vi "Set Config (Element).vi"(8 "error in (no error)":errorcluster, 10 "Config Element":refnum<class "Config Element.lvclass">, 11 "Task in":refnum<class "Task.lvclass">) -> (0 "error out":errorcluster, 3 "Task out":refnum<class "Task.lvclass">)   [LabVIEW 2020, in "Volatus.lvlib" / "Task.lvclass"]
uses:
  Task.lvclass
  lv-cdm/CDM-Config/Config Element/Config Element.lvclass
  Task.lvclass/Task.ctl
  VolatusConfig/Task/Task.lvclass
  VolatusConfig/VolatusConfigElement/VolatusConfigElement.lvclass
  C:/dev/lv20CE/relink/lv-volatus/VolatusConfig/VolatusConfigElement/VolatusConfigElement.lvclass
  C:/dev/lv20CE/relink/lv-volatus/VolatusConfig/Task/Task.lvclass
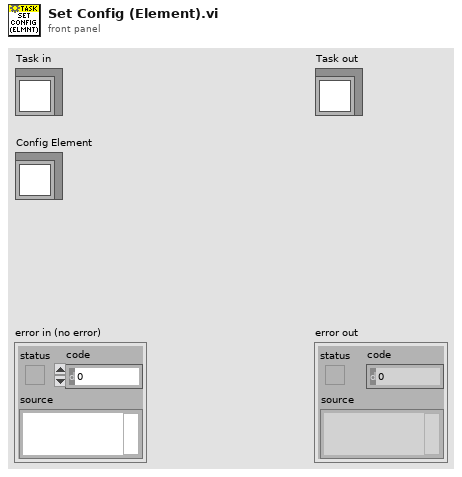
[diagram p1: front panel]
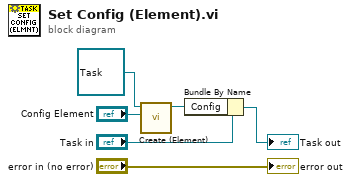
[diagram p0: block diagram]
diagram:
  n1 = call "Create (Element).vi"("Element"="Config Element", "VolatusConfigElement in"=refnum<class "Task.lvclass"> refnum ("VolatusConfig.lvlib:Task.lvclass")) -> ("VolatusConfigElement out"=w2:refnum<class "Task.lvclass">)  [unwired: 8 in, 1 out]
  n2 = Bundle By Name(cluster="Task in", "Config"=w2) -> (→"Task out":refnum<class "Task.lvclass">)
  "error out" <- "error in (no error)"
